vi "Utility Fast Comms.vi"(8 "Fast Comms":bool, 11 "Command":string) -> (3 "Fast Command":string)   [LabVIEW 2020, in "ChromTech Series I Drivers.lvlib"]
doc: "Appends a carriage return to the end of the command, indicating the end of a transmitted string. This will cause the pump to immediately respond to the received command, and may help speed communications."
uses:
  <instrlib>/RxnRover/ChromtechSeriesIDriver/ChromTech Series I Drivers.lvlib
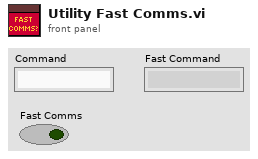
[diagram p1: front panel]
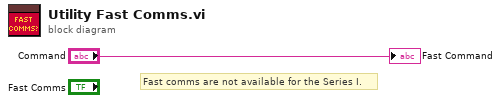
[diagram p0: block diagram]
diagram:
  # "Fast comms are not available for the Series I."
  "Fast Command" <- "Command"
